vi "Constructor.vi"(8 "error in (no error)":errorcluster, 11 "Chef in":refnum<class "Chef.lvclass">) -> (0 "error out":errorcluster, 3 "Chef out":refnum<class "Chef.lvclass">)   [LabVIEW 2011, in "Chef.lvclass"]
uses:
  Chef.lvclass
  Oven/Oven.lvclass
  Chef.lvclass/Chef.ctl
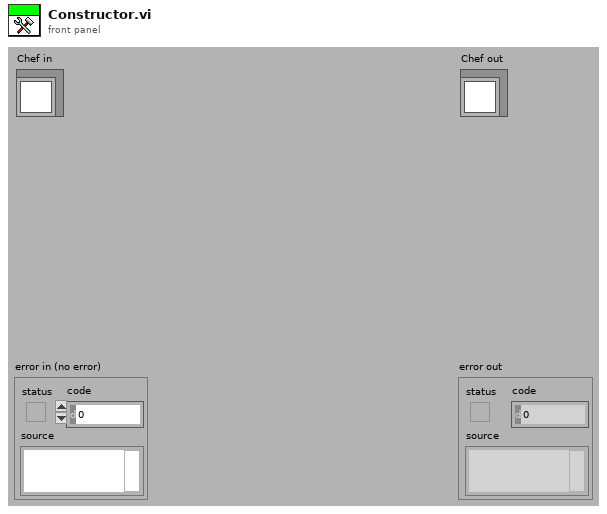
[diagram p1: front panel]
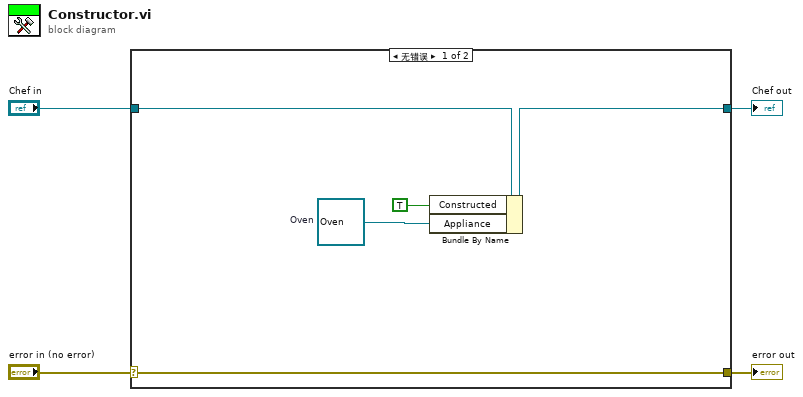
[diagram p0: block diagram]
diagram:
  n1 = case shown="无错误" "error in (no error)" {
    selector: "error in (no error)" -> [w8 w11]
    tunnel: [w8 w11] -> w3
    tunnel: [w6 w10] -> w1
    tunnel: "Chef in" -> [w9 w10]
    frame No Error {
      w5 = refnum<class "Oven.lvclass"> refnum  # Oven
      n2 = Bundle By Name(cluster=w9, "Constructed"=TRUE, "Appliance"=w5) -> (w6:refnum<class "Chef.lvclass">)
    }
    frame Error {
    }
  }
  "error out" <- w3
  "Chef out" <- w1
